vi "PLC_comm.vi"() -> ()   [LabVIEW 2017]
uses:
  <vilib>/DATA AHEAD/SP7/typedefs/PLC Type.ctl
  <vilib>/addons/database/Connection.llb/DB Tools Open Connec (String).vi
  Global/DATA LOG.vi
  <vilib>/DATA AHEAD/SP7/functions/write/write bool array.vi
  <vilib>/DATA AHEAD/SP7/functions/read/read bool array.vi
  <vilib>/DATA AHEAD/SP7/functions/read/read int array.vi
  <vilib>/DATA AHEAD/SP7/functions/read/read String.vi
  Global/Global 1.vi
  <vilib>/DATA AHEAD/SP7/functions/read/read real array.vi
  <vilib>/DATA AHEAD/SP7/functions/read/read Timeofday array.vi
  <vilib>/addons/database/NI_Database_API.lvlib
  <vilib>/DATA AHEAD/SP7/SP7.lvlib
panel:
  out "IP1 7":string
  out "PLC 7":bool
  out "IP1 6":string
  out "PLC 6":bool
  out "IP1 5":string
  out "PLC 5":bool
  out "PLC 4":bool
  out "PLC 3":bool
  out "PLC 2":bool
  out "PLC 1":bool
  out "IP1 4":string
  out "IP1 3":string
  out "IP1 2":string
  out "IP1":string
  in  "stop":bool
  out "error out":errorcluster
  in  "error in (no error)":errorcluster
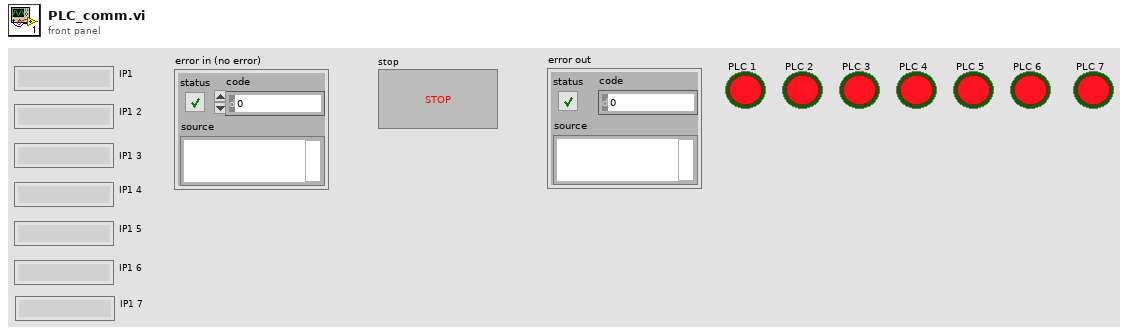
[diagram p1: front panel]
types:
  T1 = typedef "SP7.lvlib/PLC Type.ctl" = enum16{"S7 200", "S7 300/400", "S7 1200", "S7 1500", "LOGO!8"}
  T2 = typedef "NI_Database_API.lvlib/Conn ObjectReference.ctl" = refnum<k1>
  T3 = typedef "SP7.lvlib/S7 Connection.ctl" = cluster{"TCP Connection Ref":refnum<k5>, "IP address":string, "timeout ms":i32, "Connected?":bool, "PLC Type":T1, "Rack S7 400":u8, "Slot S7 400":u8, "PDU Size":u16, "connection semaphore":T4}
  T4 = typedef "Semaphore RefNum" = refnum<k1>
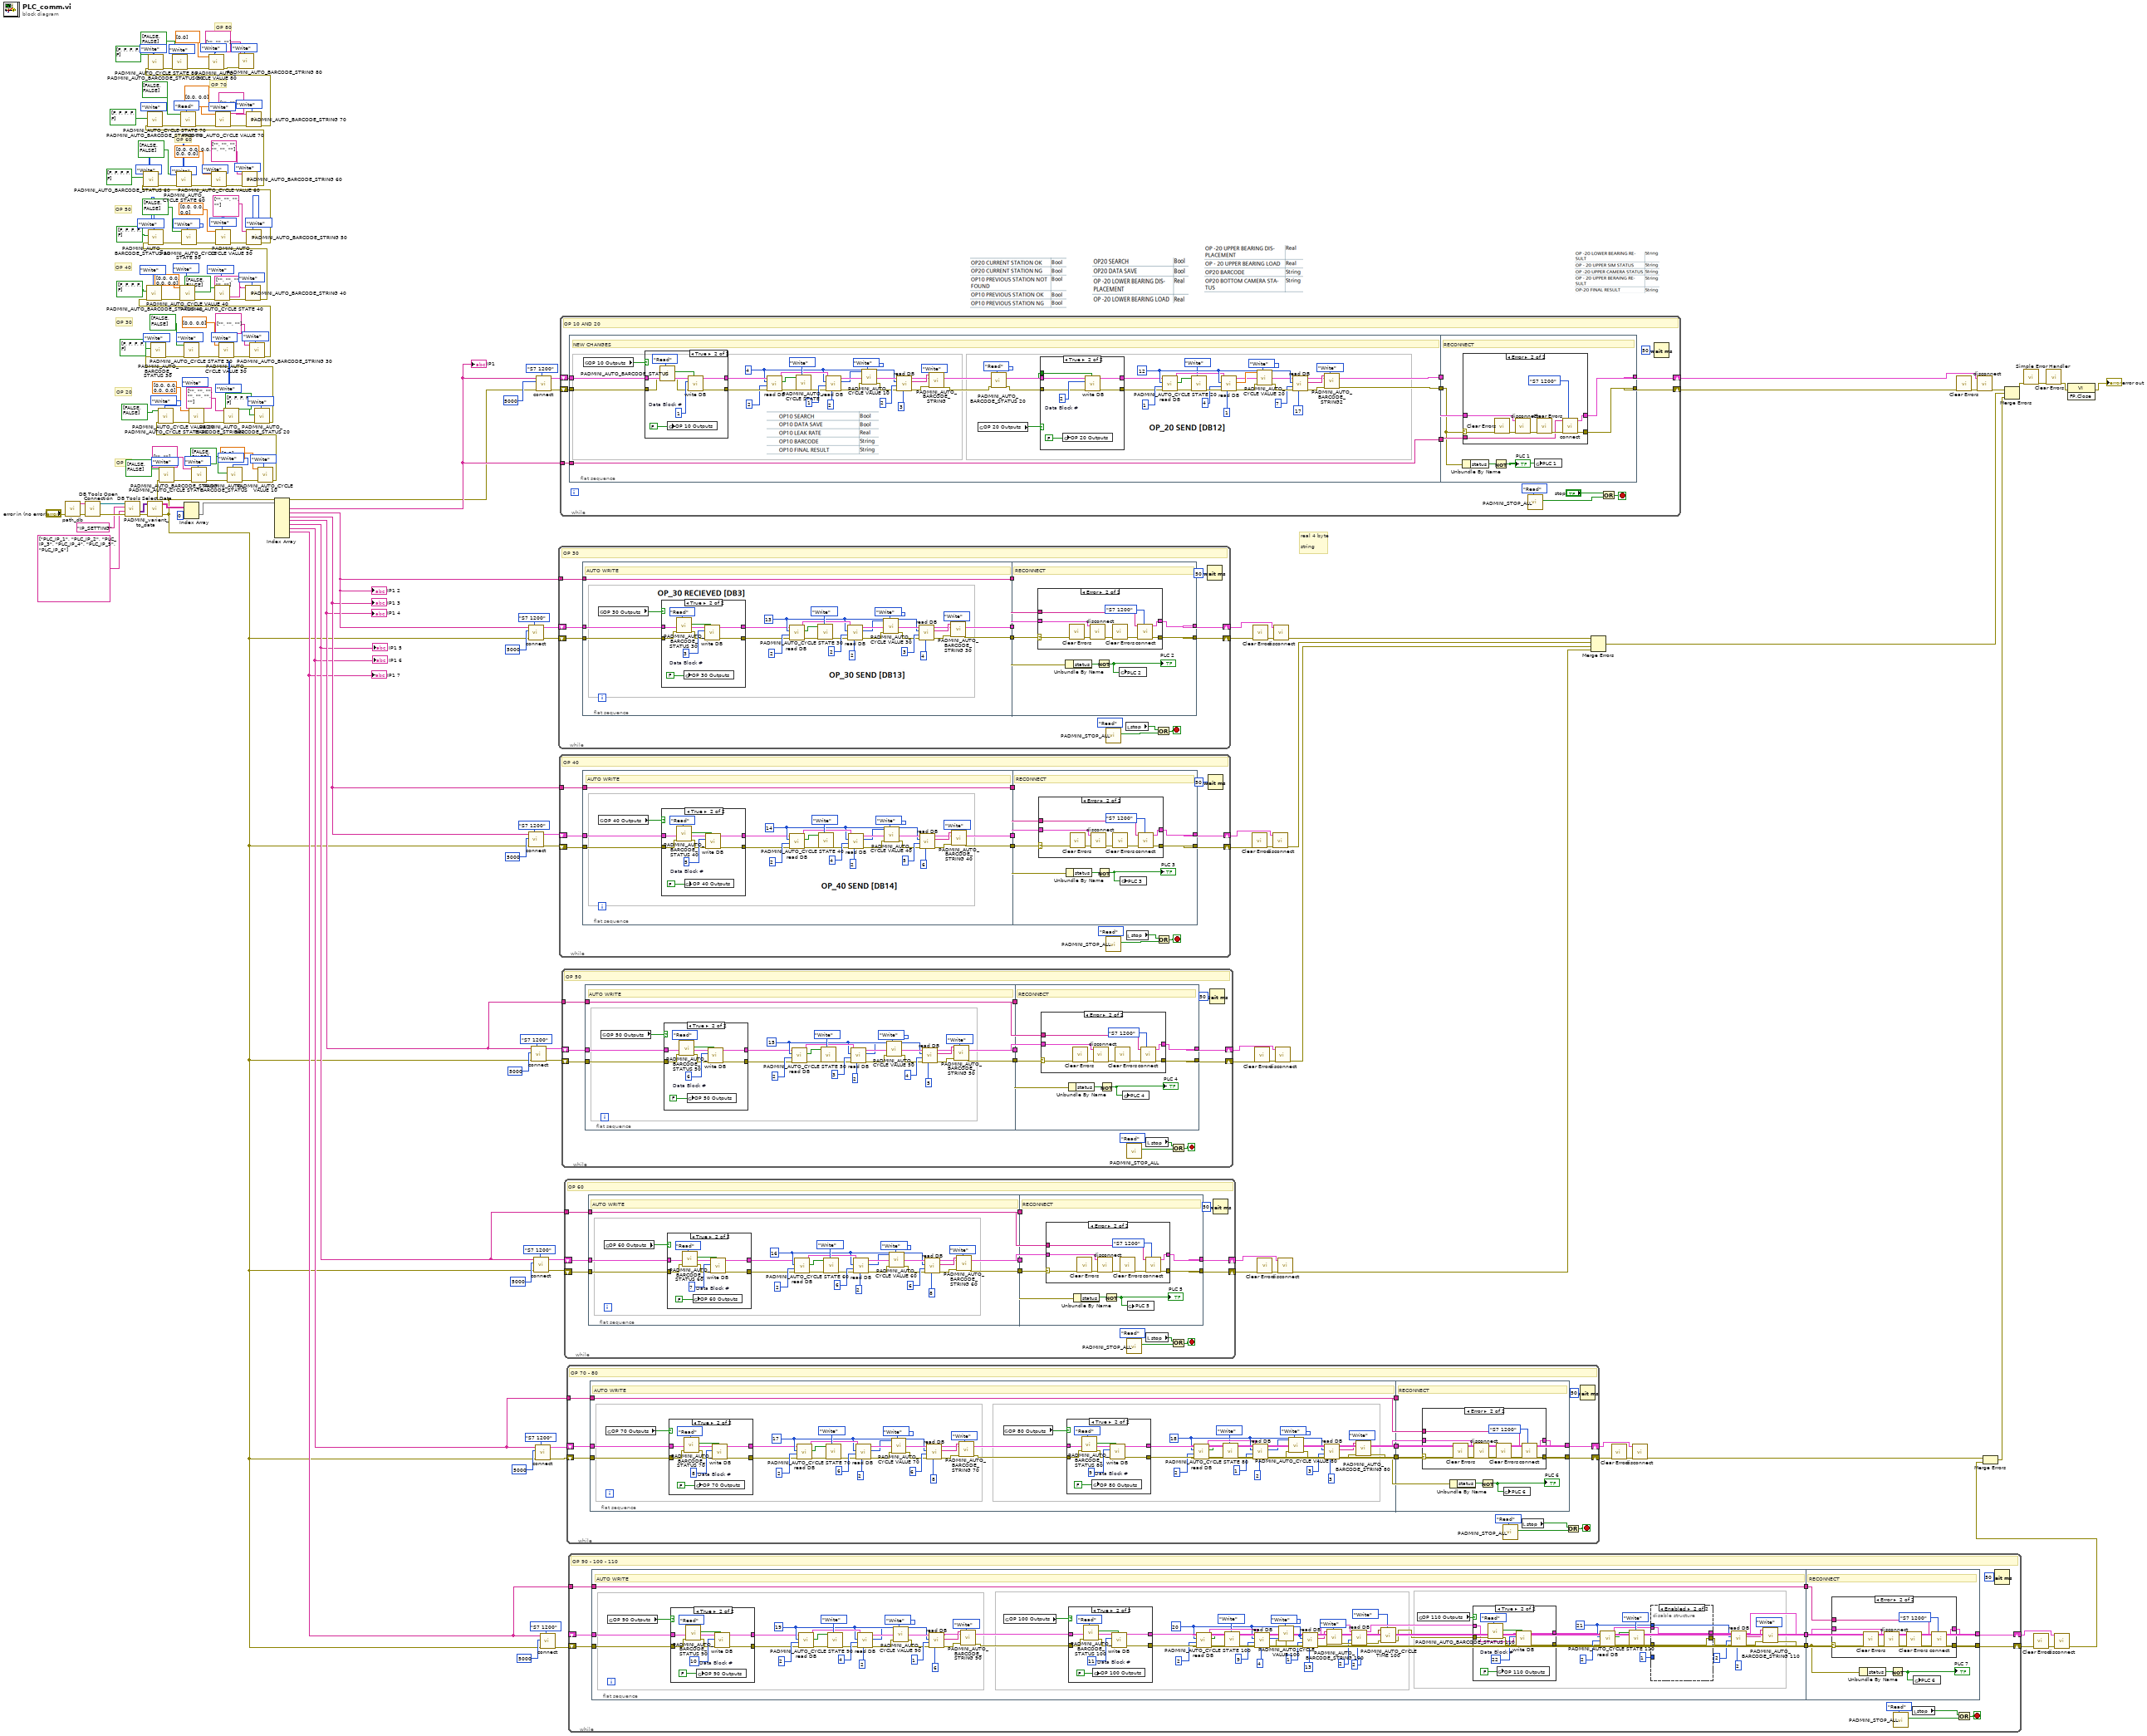
[diagram p0: block diagram]
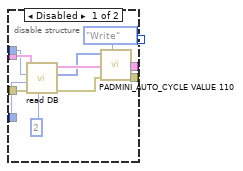
[diagram p2: hidden frame]
diagram:
  # "real 4 byte\n\nstring"
  # "OP 80"
  # "OP 70"
  # "OP 60"
  # "OP 50"
  # "OP 40"
  # "OP 30"
  # "OP 20"
  # "OP 10"
  n1 = call "path_db.vi"("error in"="error in (no error)") -> ("error out"=w171:errorcluster, "resulting string"=w176:string)  [unwired: 9 in]
  n2 = call-poly <vilib>:"DB Tools Open Connection.vi"("error in (no error)"=w171, "connection information"=w176) -> ("error out"=w175:errorcluster, "connection reference"=w174:T2)  [unwired: 6 in]
  n3 = call <vilib>:"DB Tools Select Data.vi"("error in (no error)"=w175, "columns"=string[] ["PLC_IP_1", "PLC_IP_2", "PLC_IP_3", "PLC_IP_4", "PLC_IP_5", "PLC_IP_6"], "table"="IP_SETTING", "connection reference"=w174) -> ("error out"=w173:errorcluster, "data"=w172:variant[][])  [unwired: 2 in, 1 out]
  n4 = call "PADMINI_varient_to_data.vi"("error in (no error)"=w173, "data"=w172) -> ("error out"=w7:errorcluster, "Array"=w167:string[][])  [unwired: 8 in]
  n5 = call "PADMINI_AUTO_CYCLE STATE.vi"("Enum"=enum16{"Read", "Write"}."Write", "error in (no error)"=w7, "Input"=bool[] [FALSE, FALSE]) -> ("error out"=w153:errorcluster)  [unwired: 7 in, 1 out]
  n6 = Index Array(array=w167, index (row)=0) -> (element=w166:string[])  [unwired: 1 in]
  n7 = call "PADMINI_AUTO_BARCODE_STRING.vi"("Enum"=enum16{"Read", "Write"}."Write", "error in (no error)"=w153, "Input"=string[] ["", ""]) -> ("error out"=w149:errorcluster)  [unwired: 7 in, 1 out]
  n8 = call "PADMINI_AUTO_BARCODE_STATUS.vi"("Enum"=enum16{"Read", "Write"}."Write", "error in (no error)"=w149, "I/P"=bool[] [FALSE, FALSE]) -> ("error out"=w147:errorcluster)  [unwired: 7 in, 1 out]
  n9 = call "PADMINI_AUTO_CYCLE VALUE 10.vi"("Enum"=enum16{"Read", "Write"}."Write", "error in (no error)"=w147, "Input"=dbl[] [0.0]) -> ("error out"=w141:errorcluster)  [unwired: 7 in, 1 out]
  n10 = call "PADMINI_AUTO_CYCLE STATE 20.vi"("Enum"=enum16{"Read", "Write"}."Write", "error in (no error)"=w141, "Input"=bool[] [FALSE, FALSE]) -> ("error out"=w139:errorcluster)  [unwired: 7 in, 1 out]
  n11 = call "PADMINI_AUTO_CYCLE VALUE 20.vi"("Enum"=enum16{"Read", "Write"}."Write", "error in (no error)"=w139, "Input"=dbl[] [0.0, 0.0, 0.0, 0.0]) -> ("error out"=w135:errorcluster)  [unwired: 7 in, 1 out]
  n12 = call "PADMINI_AUTO_BARCODE_STRING2.vi"("Enum"=enum16{"Read", "Write"}."Write", "error in (no error)"=w135, "Input"=string[] ["", "", "", "", "", "", ""]) -> ("error out"=w132:errorcluster)  [unwired: 7 in, 1 out]
  n13 = call "PADMINI_AUTO_BARCODE_STATUS 20.vi"("Enum"=enum16{"Read", "Write"}."Write", "error in (no error)"=w132, "I/P"=bool[] [FALSE, FALSE, FALSE, FALSE, FALSE]) -> ("error out"=w125:errorcluster)  [unwired: 7 in, 1 out]
  n14 = call "PADMINI_AUTO_BARCODE_STATUS 30.vi"("Enum"=enum16{"Read", "Write"}."Write", "error in (no error)"=w125, "I/P"=bool[] [FALSE, FALSE, FALSE, FALSE, FALSE]) -> ("error out"=w122:errorcluster)  [unwired: 7 in, 1 out]
  n15 = call "PADMINI_AUTO_CYCLE STATE 30.vi"("Enum"=enum16{"Read", "Write"}."Write", "error in (no error)"=w122, "Input"=bool[] [FALSE, FALSE]) -> ("error out"=w121:errorcluster)  [unwired: 7 in, 1 out]
  n16 = call "PADMINI_AUTO_CYCLE VALUE 30.vi"("Enum"=enum16{"Read", "Write"}."Write", "error in (no error)"=w121, "Input"=dbl[] [0.0, 0.0]) -> ("error out"=w117:errorcluster)  [unwired: 7 in, 1 out]
  n17 = call "PADMINI_AUTO_BARCODE_STRING 30.vi"("Enum"=enum16{"Read", "Write"}."Write", "error in (no error)"=w117, "Input"=string[] ["", "", ""]) -> ("error out"=w95:errorcluster)  [unwired: 7 in, 1 out]
  n18 = call "PADMINI_AUTO_BARCODE_STATUS 40.vi"("Enum"=enum16{"Read", "Write"}."Write", "error in (no error)"=w95, "I/P"=bool[] [FALSE, FALSE, FALSE, FALSE, FALSE]) -> ("error out"=w94:errorcluster)  [unwired: 7 in, 1 out]
  n19 = call "PADMINI_AUTO_CYCLE VALUE 40.vi"("Enum"=enum16{"Read", "Write"}."Write", "error in (no error)"=w94, "Input"=dbl[] [0.0, 0.0, 0.0, 0.0]) -> ("error out"=w93:errorcluster)  [unwired: 7 in, 1 out]
  n20 = call "PADMINI_AUTO_CYCLE STATE 40.vi"("Enum"=enum16{"Read", "Write"}."Write", "error in (no error)"=w93, "Input"=bool[] [FALSE, FALSE]) -> ("error out"=w92:errorcluster)  [unwired: 7 in, 1 out]
  n21 = call "PADMINI_AUTO_BARCODE_STRING 40.vi"("Enum"=enum16{"Read", "Write"}."Write", "error in (no error)"=w92, "Input"=string[] ["", "", "", "", ""]) -> ("error out"=w70:errorcluster)  [unwired: 7 in, 1 out]
  n22 = call "PADMINI_AUTO_BARCODE_STATUS 50.vi"("Enum"=enum16{"Read", "Write"}."Write", "error in (no error)"=w70, "I/P"=bool[] [FALSE, FALSE, FALSE, FALSE, FALSE]) -> ("error out"=w72:errorcluster)  [unwired: 7 in, 1 out]
  n23 = call "PADMINI_AUTO_CYCLE STATE 50.vi"("Enum"=enum16{"Read", "Write"}."Write", "error in (no error)"=w72, "Input"=bool[] [FALSE, FALSE]) -> ("error out"=w76:errorcluster)  [unwired: 7 in, 1 out]
  n24 = call "PADMINI_AUTO_CYCLE VALUE 50.vi"("Enum"=enum16{"Read", "Write"}."Write", "error in (no error)"=w76, "Input"=dbl[] [0.0, 0.0, 0.0]) -> ("error out"=w73:errorcluster)  [unwired: 7 in, 1 out]
  n25 = call "PADMINI_AUTO_BARCODE_STRING 50.vi"("Enum"=enum16{"Read", "Write"}."Write", "error in (no error)"=w73, "Input"=string[] ["", "", "", ""]) -> ("error out"=w44:errorcluster)  [unwired: 7 in, 1 out]
  n26 = call "PADMINI_AUTO_BARCODE_STATUS 60.vi"("Enum"=enum16{"Read", "Write"}."Write", "error in (no error)"=w44, "I/P"=bool[] [FALSE, FALSE, FALSE, FALSE, FALSE]) -> ("error out"=w50:errorcluster)  [unwired: 7 in, 1 out]
  n27 = call "PADMINI_AUTO_CYCLE STATE 60.vi"("Enum"=enum16{"Read", "Write"}."Write", "error in (no error)"=w50, "Input"=bool[] [FALSE, FALSE]) -> ("error out"=w52:errorcluster)  [unwired: 7 in, 1 out]
  n28 = call "PADMINI_AUTO_CYCLE VALUE 60.vi"("Enum"=enum16{"Read", "Write"}."Write", "error in (no error)"=w52, "Input"=dbl[] [0.0, 0.0, 0.0, 0.0, 0.0]) -> ("error out"=w55:errorcluster)  [unwired: 7 in, 1 out]
  n29 = call "PADMINI_AUTO_BARCODE_STRING 60.vi"("Enum"=enum16{"Read", "Write"}."Write", "error in (no error)"=w55, "Input"=string[] ["", "", "", "", "", ""]) -> ("error out"=w18:errorcluster)  [unwired: 7 in, 1 out]
  n30 = call "PADMINI_AUTO_BARCODE_STATUS 70.vi"("Enum"=enum16{"Read", "Write"}."Write", "error in (no error)"=w18, "I/P"=bool[] [FALSE, FALSE, FALSE, FALSE, FALSE]) -> ("error out"=w23:errorcluster)  [unwired: 7 in, 1 out]
  n31 = call "PADMINI_AUTO_CYCLE STATE 70.vi"("Enum"=enum16{"Read", "Write"}."Read", "error in (no error)"=w23, "Input"=bool[] [FALSE, FALSE]) -> ("error out"=w35:errorcluster)  [unwired: 7 in, 1 out]
  n32 = call "PADMINI_AUTO_CYCLE VALUE 70.vi"("Enum"=enum16{"Read", "Write"}."Write", "error in (no error)"=w35, "Input"=dbl[] [0.0, 0.0]) -> ("error out"=w32:errorcluster)  [unwired: 7 in, 1 out]
  n33 = call "PADMINI_AUTO_BARCODE_STRING 70.vi"("Enum"=enum16{"Read", "Write"}."Write", "error in (no error)"=w32, "Input"=string[] ["", ""]) -> ("error out"=w13:errorcluster)  [unwired: 7 in, 1 out]
  n34 = call "PADMINI_AUTO_BARCODE_STATUS 80.vi"("Enum"=enum16{"Read", "Write"}."Write", "error in (no error)"=w13, "I/P"=bool[] [FALSE, FALSE, FALSE, FALSE, FALSE]) -> ("error out"=w24:errorcluster)  [unwired: 7 in, 1 out]
  n35 = call "PADMINI_AUTO_CYCLE STATE 80.vi"("Enum"=enum16{"Read", "Write"}."Write", "error in (no error)"=w24, "Input"=bool[] [FALSE, FALSE]) -> ("error out"=w28:errorcluster)  [unwired: 7 in, 1 out]
  n36 = call "PADMINI_AUTO_CYCLE VALUE 80.vi"("Enum"=enum16{"Read", "Write"}."Write", "error in (no error)"=w28, "Input"=dbl[] [0.0]) -> ("error out"=w31:errorcluster)  [unwired: 7 in, 1 out]
  n37 = call "PADMINI_AUTO_BARCODE_STRING 80.vi"("Enum"=enum16{"Read", "Write"}."Write", "error in (no error)"=w31, "Input"=string[] ["", "", ""]) -> ()  [unwired: 7 in, 2 out]
  n38 = Index Array(array=w166) -> (element #1=w111:string, element #2=w112:string, element #3=w106:string, element #4=w80:string, element #5=w58:string, element #6=w9:string, element #7=w8:string)  [unwired: 8 in, 1 out]
  "IP1" <- w111
  "IP1 2" <- w112
  "IP1 3" <- w106
  "IP1 4" <- w80
  "IP1 5" <- w58
  "IP1 6" <- w9
  "IP1 7" <- w8
  n39 = call <vilib>:"connect.vi"("PLC Type"=PLC_Type."S7 1200" ("PLC Type 2"), "error in (no error)"=w7, "timeout [ms]"=5000 ("timeout [ms] 2"), "IP address"=w112) -> ("error out"=w129:errorcluster, "S7 Connection out"=w128:T3)  [unwired: 6 in]
  n40 = call <vilib>:"connect.vi"("PLC Type"=PLC_Type."S7 1200" ("PLC Type 2"), "error in (no error)"=w7, "timeout [ms]"=5000 ("timeout [ms] 2"), "IP address"=w106) -> ("error out"=w108:errorcluster, "S7 Connection out"=w107:T3)  [unwired: 6 in]
  n41 = call <vilib>:"connect.vi"("PLC Type"=PLC_Type."S7 1200" ("PLC Type 2"), "error in (no error)"=w7, "timeout [ms]"=5000 ("timeout [ms] 2"), "IP address"=w80) -> ("error out"=w83:errorcluster, "S7 Connection out"=w84:T3)  [unwired: 6 in]
  n42 = call <vilib>:"connect.vi"("PLC Type"=PLC_Type."S7 1200" ("PLC Type 2"), "error in (no error)"=w7, "timeout [ms]"=5000 ("timeout [ms] 2"), "IP address"=w58) -> ("error out"=w63:errorcluster, "S7 Connection out"=w62:T3)  [unwired: 6 in]
  n43 = call <vilib>:"connect.vi"("PLC Type"=PLC_Type."S7 1200" ("PLC Type 2"), "error in (no error)"=w7, "timeout [ms]"=5000 ("timeout [ms] 2"), "IP address"=w9) -> ("error out"=w41:errorcluster, "S7 Connection out"=w40:T3)  [unwired: 6 in]
  n44 = call <vilib>:"connect.vi"("PLC Type"=PLC_Type."S7 1200" ("PLC Type 2"), "error in (no error)"=w7, "timeout [ms]"=5000, "IP address"=w111) -> ("error out"=w157:errorcluster, "S7 Connection out"=w156:T3)  [unwired: 6 in]
  n45 = call <vilib>:"connect.vi"("PLC Type"=PLC_Type."S7 1200" ("PLC Type 2"), "error in (no error)"=w7, "timeout [ms]"=5000 ("timeout [ms] 2"), "IP address"=w8) -> ("error out"=w10:errorcluster)  [unwired: 6 in, 1 out]
  n46 = while {
    shift-right: [w179] -> w114
    shift-left: w128 -> [w189]
    shift-right: [w187] -> w113
    shift-left: w129 -> [w188]
    tunnel: w112 -> [w178]
    stop <- w181 stop-if-true
    # "OP 30"
    n47 = flat-sequence {
      tunnel: [w192] -> w185
      tunnel: [w191] -> w180
      tunnel: w188 -> [w216]
      tunnel: w189 -> [w215]
      tunnel: w178 -> [w190]
      tunnel: [w190] -> w177
      tunnel: [w230] -> w187
      tunnel: [w229] -> w179
      tunnel: w185 -> [w232]
      tunnel: w180 -> [w231]
      tunnel: w177 -> [w228]
      frame #0 {
        w205 = u16 13 ("Data Block #")
        # "AUTO WRITE"
        n48 = global read "DATA LOG.vi" "OP 30 Outputs"() -> (w214:bool)
        n49 = case shown="True" w214 {
          tunnel: w215 -> [w217 w226]
          tunnel: [w218 w225] -> w193
          tunnel: [w217 w224] -> w194
          tunnel: w216 -> [w218 w221]
          frame False {
          }
          frame True {
            w227 = u16 3  # Data Block #
            n50 = call "PADMINI_AUTO_BARCODE_STATUS 30.vi"("Enum"=enum16{"Read", "Write"}."Read", "error in (no error)"=w221) -> ("error out"=w220:errorcluster, "O/P"=w222:bool[])  [unwired: 8 in]
            n51 = global write "DATA LOG.vi" "OP 30 Outputs"(FALSE) -> ()
            n52 = call-poly <vilib>:"write DB.vi"("BOOL input array [byte]"=w222, "error in (no error)"=w220, "Data Block #"=w227, "S7 Connection in"=w226) -> ("error out"=w225:errorcluster, "S7 Connection out"=w224:T3)  [unwired: 4 in, 2 out]
          }
        }
        n53 = call-poly <vilib>:"read DB.vi"("error in (no error)"=w193, "Items # [byte]"=u16 2, "Data Block #"=w205, "S7 Connection in"=w194) -> ("error out"=w212:errorcluster, "BOOL result array  [byte]"=w210:bool[], "S7 Connection out"=w207:T3)  [unwired: 5 in]
        n54 = call "PADMINI_AUTO_CYCLE STATE 30.vi"("Enum"=enum16{"Read", "Write"}."Write", "error in (no error)"=w212, "Input"=w210) -> ("error out"=w208:errorcluster)  [unwired: 7 in, 1 out]
        n55 = call-poly <vilib>:"read DB.vi"("Item offset [byte]"=u32 2, "error in (no error)"=w208, "items #"=u16 2 ("Items # [byte]"), "Data Block #"=w205, "S7 Connection in"=w207) -> ("error out"=w197:errorcluster, "Int result array"=w195:i16[], "S7 Connection out"=w206:T3)  [unwired: 4 in]
        n56 = call "PADMINI_AUTO_CYCLE VALUE 30.vi"("Enum"=enum16{"Read", "Write"}."Write", "error in (no error)"=w197, "Input"=w195) -> ("error out"=w196:errorcluster)  [unwired: 7 in, 1 out]
        n57 = call-poly <vilib>:"read DB.vi"("Item offset [byte]"=u32 4, "error in (no error)"=w196, "items #"=u16 3 ("Items # [byte]"), "Data Block #"=w205, "S7 Connection in"=w206) -> ("error out"=w201:errorcluster, "STRING result Array"=w202:string[], "S7 Connection out"=w192:T3)  [unwired: 3 in, 1 out]
        n58 = call "PADMINI_AUTO_BARCODE_STRING 30.vi"("Enum"=enum16{"Read", "Write"}."Write", "error in (no error)"=w201, "Input"=w202) -> ("error out"=w191:errorcluster)  [unwired: 7 in, 1 out]
      }
      frame #1 {
        # "RECONNECT"
        n59 = case shown="Error" w231 {
          selector: w231 -> [w236 w244]
          tunnel: [w235 w241] -> w229
          tunnel: [w236 w242] -> w230
          tunnel: w232 -> [w235 w238]
          tunnel: w228 -> [_ w237]
          frame No Error {
          }
          frame Error {
            n60 = call <vilib>:"Clear Errors.vi"("error in (no error)"=w244) -> ("error out"=w245:errorcluster)  [unwired: 5 in, 1 out]
            n61 = call <vilib>:"disconnect.vi"("error in (no error)"=w245, "S7 Connection in"=w238) -> ("error out"=w243:errorcluster)  [unwired: 8 in, 1 out]
            n62 = call <vilib>:"Clear Errors.vi"("error in (no error)"=w243) -> ("error out"=w240:errorcluster)  [unwired: 5 in, 1 out]
            n63 = call <vilib>:"connect.vi"("PLC Type"=PLC_Type."S7 1200" ("PLC Type 2"), "error in (no error)"=w240, "IP address"=w237) -> ("error out"=w242:errorcluster, "S7 Connection out"=w241:T3)  [unwired: 7 in]
          }
        }
        n64 = Unbundle By Name(w231) -> ("status"=w234:bool)
        n65 = Not(x=w234) -> (.not. x?=w233:bool)
        "PLC 2" <- w233
        n66 = global write "Global 1.vi" "PLC 2"(w233) -> ()
      }
    }
    n67 = call "PADMINI_STOP_ALL.vi"("Enum"=enum16{"Read", "Write"}."Read") -> ("Boolean 2"=w183:bool)  [unwired: 9 in, 1 out]
    n68 = local read "stop"() -> (w182:bool)
    n69 = Or(x=w182, y=w183) -> (x .or. y?=w181:bool)
    n70 = Wait (ms)(milliseconds to wait=u32 50) -> ()  [unwired: 1 out]
  }
  n71 = while {
    shift-right: [w248] -> w103
    shift-left: w107 -> [w258]
    shift-right: [w256] -> w104
    shift-left: w108 -> [w257]
    tunnel: w106 -> [w247]
    stop <- w250 stop-if-true
    # "OP 40"
    n72 = flat-sequence {
      tunnel: [w261] -> w254
      tunnel: [w260] -> w249
      tunnel: w257 -> [w285]
      tunnel: w258 -> [w284]
      tunnel: w247 -> [w259]
      tunnel: [w259] -> w246
      tunnel: [w299] -> w256
      tunnel: [w298] -> w248
      tunnel: w254 -> [w301]
      tunnel: w249 -> [w300]
      tunnel: w246 -> [w297]
      frame #0 {
        w274 = u16 14 ("Data Block #")
        # "AUTO WRITE"
        n73 = global read "DATA LOG.vi" "OP 40 Outputs"() -> (w283:bool)
        n74 = case shown="True" w283 {
          tunnel: w284 -> [w286 w295]
          tunnel: [w287 w294] -> w262
          tunnel: [w286 w293] -> w263
          tunnel: w285 -> [w287 w290]
          frame False {
          }
          frame True {
            w296 = u16 5  # Data Block #
            n75 = call "PADMINI_AUTO_BARCODE_STATUS 40.vi"("Enum"=enum16{"Read", "Write"}."Read", "error in (no error)"=w290) -> ("error out"=w289:errorcluster, "O/P"=w291:bool[])  [unwired: 8 in]
            n76 = global write "DATA LOG.vi" "OP 40 Outputs"(FALSE) -> ()
            n77 = call-poly <vilib>:"write DB.vi"("BOOL input array [byte]"=w291, "error in (no error)"=w289, "Data Block #"=w296, "S7 Connection in"=w295) -> ("error out"=w294:errorcluster, "S7 Connection out"=w293:T3)  [unwired: 4 in, 2 out]
          }
        }
        n78 = call-poly <vilib>:"read DB.vi"("error in (no error)"=w262, "Items # [byte]"=u16 2, "Data Block #"=w274, "S7 Connection in"=w263) -> ("error out"=w281:errorcluster, "BOOL result array  [byte]"=w279:bool[], "S7 Connection out"=w276:T3)  [unwired: 5 in]
        n79 = call "PADMINI_AUTO_CYCLE STATE 40.vi"("Enum"=enum16{"Read", "Write"}."Write", "error in (no error)"=w281, "Input"=w279) -> ("error out"=w277:errorcluster)  [unwired: 7 in, 1 out]
        n80 = call-poly <vilib>:"read DB.vi"("Item offset [byte]"=u32 2, "error in (no error)"=w277, "items #"=u16 4 ("Items # [byte]"), "Data Block #"=w274, "S7 Connection in"=w276) -> ("error out"=w266:errorcluster, "Int result array"=w264:i16[], "S7 Connection out"=w275:T3)  [unwired: 4 in]
        n81 = call "PADMINI_AUTO_CYCLE VALUE 40.vi"("Enum"=enum16{"Read", "Write"}."Write", "error in (no error)"=w266, "Input"=w264) -> ("error out"=w265:errorcluster)  [unwired: 7 in, 1 out]
        n82 = call-poly <vilib>:"read DB.vi"("Item offset [byte]"=u32 6, "error in (no error)"=w265, "items #"=u16 5 ("Items # [byte]"), "Data Block #"=w274, "S7 Connection in"=w275) -> ("error out"=w270:errorcluster, "STRING result Array"=w271:string[], "S7 Connection out"=w261:T3)  [unwired: 3 in, 1 out]
        n83 = call "PADMINI_AUTO_BARCODE_STRING 40.vi"("Enum"=enum16{"Read", "Write"}."Write", "error in (no error)"=w270, "Input"=w271) -> ("error out"=w260:errorcluster)  [unwired: 7 in, 1 out]
      }
      frame #1 {
        # "RECONNECT"
        n84 = case shown="Error" w300 {
          selector: w300 -> [w305 w313]
          tunnel: [w304 w310] -> w298
          tunnel: [w305 w311] -> w299
          tunnel: w301 -> [w304 w307]
          tunnel: w297 -> [_ w306]
          frame No Error {
          }
          frame Error {
            n85 = call <vilib>:"Clear Errors.vi"("error in (no error)"=w313) -> ("error out"=w314:errorcluster)  [unwired: 5 in, 1 out]
            n86 = call <vilib>:"disconnect.vi"("error in (no error)"=w314, "S7 Connection in"=w307) -> ("error out"=w312:errorcluster)  [unwired: 8 in, 1 out]
            n87 = call <vilib>:"Clear Errors.vi"("error in (no error)"=w312) -> ("error out"=w309:errorcluster)  [unwired: 5 in, 1 out]
            n88 = call <vilib>:"connect.vi"("PLC Type"=PLC_Type."S7 1200" ("PLC Type 2"), "error in (no error)"=w309, "IP address"=w306) -> ("error out"=w311:errorcluster, "S7 Connection out"=w310:T3)  [unwired: 7 in]
          }
        }
        n89 = Unbundle By Name(w300) -> ("status"=w303:bool)
        n90 = Not(x=w303) -> (.not. x?=w302:bool)
        "PLC 3" <- w302
        n91 = global write "Global 1.vi" "PLC 3"(w302) -> ()
      }
    }
    n92 = call "PADMINI_STOP_ALL.vi"("Enum"=enum16{"Read", "Write"}."Read") -> ("Boolean 2"=w252:bool)  [unwired: 9 in, 1 out]
    n93 = local read "stop"() -> (w251:bool)
    n94 = Or(x=w251, y=w252) -> (x .or. y?=w250:bool)
    n95 = Wait (ms)(milliseconds to wait=u32 50) -> ()  [unwired: 1 out]
  }
  n96 = while {
    shift-right: [w317] -> w144
    shift-left: w156 -> [w327]
    shift-right: [w325] -> w160
    shift-left: w157 -> [w326]
    tunnel: w111 -> [w315]
    stop <- w320 stop-if-true
    # "OP 10 AND 20"
    n97 = flat-sequence {
      tunnel: [w330] -> w319
      tunnel: [w329] -> w318
      tunnel: w326 -> [w363]
      tunnel: w327 -> [w380]
      tunnel: [w328] -> w316
      tunnel: w315 -> [w328]
      tunnel: [w405] -> w325
      tunnel: [w404] -> w317
      tunnel: w319 -> [w406]
      tunnel: w318 -> [w402]
      tunnel: w316 -> [w403]
      frame #0 {
        w345 = u16 12 ("Data Block #")
        w370 = u16 4 ("Data Block #")
        # "NEW CHANGES"
        n98 = global read "DATA LOG.vi" "OP 10 Outputs"() -> (w362:bool)
        n99 = case shown="True" w362 {
          tunnel: w380 -> [w391 w400]
          tunnel: [w392 w399] -> w379
          tunnel: [w391 w398] -> w377
          tunnel: w363 -> [w392 w395]
          frame False {
          }
          frame True {
            w401 = u16 1  # Data Block #
            n100 = call "PADMINI_AUTO_BARCODE_STATUS.vi"("Enum"=enum16{"Read", "Write"}."Read", "error in (no error)"=w395) -> ("error out"=w394:errorcluster, "O/P"=w396:bool[])  [unwired: 8 in]
            n101 = global write "DATA LOG.vi" "OP 10 Outputs"(FALSE) -> ()
            n102 = call-poly <vilib>:"write DB.vi"("BOOL input array [byte]"=w396, "error in (no error)"=w394, "Data Block #"=w401, "S7 Connection in"=w400) -> ("error out"=w399:errorcluster, "S7 Connection out"=w398:T3)  [unwired: 4 in, 2 out]
          }
        }
        n103 = call-poly <vilib>:"read DB.vi"("error in (no error)"=w379, "Items # [byte]"=u16 2, "Data Block #"=w370, "S7 Connection in"=w377) -> ("error out"=w378:errorcluster, "BOOL result array  [byte]"=w375:bool[], "S7 Connection out"=w372:T3)  [unwired: 5 in]
        n104 = call "PADMINI_AUTO_CYCLE STATE.vi"("Enum"=enum16{"Read", "Write"}."Write", "error in (no error)"=w378, "Input"=w375) -> ("error out"=w373:errorcluster)  [unwired: 7 in, 1 out]
        n105 = call-poly <vilib>:"read DB.vi"("Item offset [byte]"=u32 2, "error in (no error)"=w373, "items #"=u16 1 ("Items # [byte]"), "Data Block #"=w370, "S7 Connection in"=w372) -> ("error out"=w360:errorcluster, "Int result array"=w358:i16[], "S7 Connection out"=w371:T3)  [unwired: 4 in]
        n106 = call "PADMINI_AUTO_CYCLE VALUE 10.vi"("Enum"=enum16{"Read", "Write"}."Write", "error in (no error)"=w360, "Input"=w358) -> ("error out"=w359:errorcluster)  [unwired: 7 in, 1 out]
        n107 = call-poly <vilib>:"read DB.vi"("Item offset [byte]"=u32 3, "error in (no error)"=w359, "items #"=u16 2 ("Items # [byte]"), "Data Block #"=w370, "S7 Connection in"=w371) -> ("error out"=w366:errorcluster, "STRING result Array"=w367:string[], "S7 Connection out"=w357:T3)  [unwired: 3 in, 1 out]
        n108 = call "PADMINI_AUTO_BARCODE_STRING.vi"("Enum"=enum16{"Read", "Write"}."Write", "error in (no error)"=w366, "Input"=w367) -> ("error out"=w333:errorcluster)  [unwired: 7 in, 1 out]
        n109 = global read "DATA LOG.vi" "OP 20 Outputs"() -> (w356:bool)
        n110 = call "PADMINI_AUTO_BARCODE_STATUS 20.vi"("Enum"=enum16{"Read", "Write"}."Read", "error in (no error)"=w333) -> ("error out"=w332:errorcluster, "O/P"=w331:bool[])  [unwired: 8 in]
        n111 = case shown="True" w356 {
          tunnel: w357 -> [w382 w386]
          tunnel: [w383 w389] -> w336
          tunnel: [w382 w388] -> w335
          tunnel: w332 -> [w383 w385]
          tunnel: w331 -> [_ w384]
          frame False {
          }
          frame True {
            w390 = u16 2  # Data Block #
            n112 = global write "DATA LOG.vi" "OP 20 Outputs"(FALSE) -> ()
            n113 = call-poly <vilib>:"write DB.vi"("BOOL input array [byte]"=w384, "error in (no error)"=w385, "Data Block #"=w390, "S7 Connection in"=w386) -> ("error out"=w389:errorcluster, "S7 Connection out"=w388:T3)  [unwired: 4 in, 2 out]
          }
        }
        n114 = call-poly <vilib>:"read DB.vi"("error in (no error)"=w336, "Items # [byte]"=u16 1, "Data Block #"=w345, "S7 Connection in"=w335) -> ("error out"=w338:errorcluster, "BOOL result array  [byte]"=w340:bool[], "S7 Connection out"=w343:T3)  [unwired: 5 in]
        n115 = call "PADMINI_AUTO_CYCLE STATE 20.vi"("Enum"=enum16{"Read", "Write"}."Write", "error in (no error)"=w338, "Input"=w340) -> ("error out"=w342:errorcluster)  [unwired: 7 in, 1 out]
        n116 = call-poly <vilib>:"read DB.vi"("Item offset [byte]"=u32 1, "error in (no error)"=w342, "items #"=u16 4 ("Items # [byte]"), "Data Block #"=w345, "S7 Connection in"=w343) -> ("error out"=w353:errorcluster, "REAL result array"=w355:sgl[], "S7 Connection out"=w344:T3)  [unwired: 4 in]
        n117 = call "PADMINI_AUTO_CYCLE VALUE 20.vi"("Enum"=enum16{"Read", "Write"}."Write", "error in (no error)"=w353, "Input"=w355) -> ("error out"=w354:errorcluster)  [unwired: 7 in, 1 out]
        n118 = call-poly <vilib>:"read DB.vi"("Item offset [byte]"=u32 17, "error in (no error)"=w354, "items #"=u16 7 ("Items # [byte]"), "Data Block #"=w345, "S7 Connection in"=w344) -> ("error out"=w349:errorcluster, "STRING result Array"=w348:string[], "S7 Connection out"=w330:T3)  [unwired: 3 in, 1 out]
        n119 = call "PADMINI_AUTO_BARCODE_STRING2.vi"("Enum"=enum16{"Read", "Write"}."Write", "error in (no error)"=w349, "Input"=w348) -> ("error out"=w329:errorcluster)  [unwired: 7 in, 1 out]
      }
      frame #1 {
        # "RECONNECT"
        n120 = Unbundle By Name(w402) -> ("status"=w408:bool)
        n121 = case shown="Error" w402 {
          selector: w402 -> [w410 w418]
          tunnel: [w409 w415] -> w404
          tunnel: [w410 w416] -> w405
          tunnel: w406 -> [w409 w412]
          tunnel: w403 -> [_ w411]
          frame No Error {
          }
          frame Error {
            n122 = call <vilib>:"Clear Errors.vi"("error in (no error)"=w418) -> ("error out"=w419:errorcluster)  [unwired: 5 in, 1 out]
            n123 = call <vilib>:"disconnect.vi"("error in (no error)"=w419, "S7 Connection in"=w412) -> ("error out"=w417:errorcluster)  [unwired: 8 in, 1 out]
            n124 = call <vilib>:"Clear Errors.vi"("error in (no error)"=w417) -> ("error out"=w414:errorcluster)  [unwired: 5 in, 1 out]
            n125 = call <vilib>:"connect.vi"("PLC Type"=PLC_Type."S7 1200" ("PLC Type 2"), "error in (no error)"=w414, "IP address"=w411) -> ("error out"=w416:errorcluster, "S7 Connection out"=w415:T3)  [unwired: 7 in]
          }
        }
        n126 = Not(x=w408) -> (.not. x?=w407:bool)
        "PLC 1" <- w407
        n127 = global write "Global 1.vi" "PLC 1"(w407) -> ()
      }
    }
    n128 = call "PADMINI_STOP_ALL.vi"("Enum"=enum16{"Read", "Write"}."Read") -> ("Boolean 2"=w322:bool)  [unwired: 9 in, 1 out]
    n129 = Or(x="stop", y=w322) -> (x .or. y?=w320:bool)
    n130 = Wait (ms)(milliseconds to wait=u32 50) -> ()  [unwired: 1 out]
  }
  n131 = while {
    shift-right: [w422] -> w87
    shift-left: w84 -> [w432]
    shift-right: [w430] -> w86
    shift-left: w83 -> [w431]
    tunnel: w80 -> [w421]
    stop <- w424 stop-if-true
    # "OP 50"
    n132 = flat-sequence {
      tunnel: [w435] -> w428
      tunnel: [w434] -> w423
      tunnel: w431 -> [w459]
      tunnel: w432 -> [w458]
      tunnel: w421 -> [w433]
      tunnel: [w433] -> w420
      tunnel: [w473] -> w430
      tunnel: [w472] -> w422
      tunnel: w428 -> [w475]
      tunnel: w423 -> [w474]
      tunnel: w420 -> [w471]
      frame #0 {
        w448 = u16 15 ("Data Block #")
        # "AUTO WRITE"
        n133 = global read "DATA LOG.vi" "OP 50 Outputs"() -> (w457:bool)
        n134 = case shown="True" w457 {
          tunnel: w458 -> [w460 w469]
          tunnel: [w461 w468] -> w436
          tunnel: [w460 w467] -> w437
          tunnel: w459 -> [w461 w464]
          frame False {
          }
          frame True {
            w470 = u16 6  # Data Block #
            n135 = call "PADMINI_AUTO_BARCODE_STATUS 50.vi"("Enum"=enum16{"Read", "Write"}."Read", "error in (no error)"=w464) -> ("error out"=w463:errorcluster, "O/P"=w465:bool[])  [unwired: 8 in]
            n136 = global write "DATA LOG.vi" "OP 50 Outputs"(FALSE) -> ()
            n137 = call-poly <vilib>:"write DB.vi"("BOOL input array [byte]"=w465, "error in (no error)"=w463, "Data Block #"=w470, "S7 Connection in"=w469) -> ("error out"=w468:errorcluster, "S7 Connection out"=w467:T3)  [unwired: 4 in, 2 out]
          }
        }
        n138 = call-poly <vilib>:"read DB.vi"("error in (no error)"=w436, "Items # [byte]"=u16 2, "Data Block #"=w448, "S7 Connection in"=w437) -> ("error out"=w455:errorcluster, "BOOL result array  [byte]"=w453:bool[], "S7 Connection out"=w450:T3)  [unwired: 5 in]
        n139 = call "PADMINI_AUTO_CYCLE STATE 50.vi"("Enum"=enum16{"Read", "Write"}."Write", "error in (no error)"=w455, "Input"=w453) -> ("error out"=w451:errorcluster)  [unwired: 7 in, 1 out]
        n140 = call-poly <vilib>:"read DB.vi"("Item offset [byte]"=u32 2, "error in (no error)"=w451, "items #"=u16 3 ("Items # [byte]"), "Data Block #"=w448, "S7 Connection in"=w450) -> ("error out"=w440:errorcluster, "Int result array"=w438:i16[], "S7 Connection out"=w449:T3)  [unwired: 4 in]
        n141 = call "PADMINI_AUTO_CYCLE VALUE 50.vi"("Enum"=enum16{"Read", "Write"}."Write", "error in (no error)"=w440, "Input"=w438) -> ("error out"=w439:errorcluster)  [unwired: 7 in, 1 out]
        n142 = call-poly <vilib>:"read DB.vi"("Item offset [byte]"=u32 5, "error in (no error)"=w439, "items #"=u16 4 ("Items # [byte]"), "Data Block #"=w448, "S7 Connection in"=w449) -> ("error out"=w444:errorcluster, "STRING result Array"=w445:string[], "S7 Connection out"=w435:T3)  [unwired: 3 in, 1 out]
        n143 = call "PADMINI_AUTO_BARCODE_STRING 50.vi"("Enum"=enum16{"Read", "Write"}."Write", "error in (no error)"=w444, "Input"=w445) -> ("error out"=w434:errorcluster)  [unwired: 7 in, 1 out]
      }
      frame #1 {
        # "RECONNECT"
        n144 = case shown="Error" w474 {
          selector: w474 -> [w479 w487]
          tunnel: [w478 w484] -> w472
          tunnel: [w479 w485] -> w473
          tunnel: w475 -> [w478 w481]
          tunnel: w471 -> [_ w480]
          frame No Error {
          }
          frame Error {
            n145 = call <vilib>:"Clear Errors.vi"("error in (no error)"=w487) -> ("error out"=w488:errorcluster)  [unwired: 5 in, 1 out]
            n146 = call <vilib>:"disconnect.vi"("error in (no error)"=w488, "S7 Connection in"=w481) -> ("error out"=w486:errorcluster)  [unwired: 8 in, 1 out]
            n147 = call <vilib>:"Clear Errors.vi"("error in (no error)"=w486) -> ("error out"=w483:errorcluster)  [unwired: 5 in, 1 out]
            n148 = call <vilib>:"connect.vi"("PLC Type"=PLC_Type."S7 1200" ("PLC Type 2"), "error in (no error)"=w483, "IP address"=w480) -> ("error out"=w485:errorcluster, "S7 Connection out"=w484:T3)  [unwired: 7 in]
          }
        }
        n149 = Unbundle By Name(w474) -> ("status"=w477:bool)
        n150 = Not(x=w477) -> (.not. x?=w476:bool)
        "PLC 4" <- w476
        n151 = global write "Global 1.vi" "PLC 4"(w476) -> ()
      }
    }
    n152 = call "PADMINI_STOP_ALL.vi"("Enum"=enum16{"Read", "Write"}."Read") -> ("Boolean 2"=w426:bool)  [unwired: 9 in, 1 out]
    n153 = local read "stop"() -> (w425:bool)
    n154 = Or(x=w425, y=w426) -> (x .or. y?=w424:bool)
    n155 = Wait (ms)(milliseconds to wait=u32 50) -> ()  [unwired: 1 out]
  }
  n156 = while {
    shift-right: [w491] -> w59
    shift-left: w62 -> [w501]
    shift-right: [w499] -> w60
    shift-left: w63 -> [w500]
    tunnel: w58 -> [w490]
    stop <- w493 stop-if-true
    # "OP 60"
    n157 = flat-sequence {
      tunnel: [w504] -> w497
      tunnel: [w503] -> w492
      tunnel: w500 -> [w528]
      tunnel: w501 -> [w527]
      tunnel: w490 -> [w502]
      tunnel: [w502] -> w489
      tunnel: [w542] -> w499
      tunnel: [w541] -> w491
      tunnel: w497 -> [w544]
      tunnel: w492 -> [w543]
      tunnel: w489 -> [w540]
      frame #0 {
        w517 = u16 16 ("Data Block #")
        # "AUTO WRITE"
        n158 = global read "DATA LOG.vi" "OP 60 Outputs"() -> (w526:bool)
        n159 = case shown="True" w526 {
          tunnel: w527 -> [w529 w538]
          tunnel: [w530 w537] -> w505
          tunnel: [w529 w536] -> w506
          tunnel: w528 -> [w530 w533]
          frame False {
          }
          frame True {
            w539 = u16 7  # Data Block #
            n160 = call "PADMINI_AUTO_BARCODE_STATUS 60.vi"("Enum"=enum16{"Read", "Write"}."Read", "error in (no error)"=w533) -> ("error out"=w532:errorcluster, "O/P"=w534:bool[])  [unwired: 8 in]
            n161 = global write "DATA LOG.vi" "OP 60 Outputs"(FALSE) -> ()
            n162 = call-poly <vilib>:"write DB.vi"("BOOL input array [byte]"=w534, "error in (no error)"=w532, "Data Block #"=w539, "S7 Connection in"=w538) -> ("error out"=w537:errorcluster, "S7 Connection out"=w536:T3)  [unwired: 4 in, 2 out]
          }
        }
        n163 = call-poly <vilib>:"read DB.vi"("error in (no error)"=w505, "Items # [byte]"=u16 2, "Data Block #"=w517, "S7 Connection in"=w506) -> ("error out"=w524:errorcluster, "BOOL result array  [byte]"=w522:bool[], "S7 Connection out"=w519:T3)  [unwired: 5 in]
        n164 = call "PADMINI_AUTO_CYCLE STATE 60.vi"("Enum"=enum16{"Read", "Write"}."Write", "error in (no error)"=w524, "Input"=w522) -> ("error out"=w520:errorcluster)  [unwired: 7 in, 1 out]
        n165 = call-poly <vilib>:"read DB.vi"("Item offset [byte]"=u32 2, "error in (no error)"=w520, "items #"=u16 6 ("Items # [byte]"), "Data Block #"=w517, "S7 Connection in"=w519) -> ("error out"=w509:errorcluster, "Int result array"=w507:i16[], "S7 Connection out"=w518:T3)  [unwired: 4 in]
        n166 = call "PADMINI_AUTO_CYCLE VALUE 60.vi"("Enum"=enum16{"Read", "Write"}."Write", "error in (no error)"=w509, "Input"=w507) -> ("error out"=w508:errorcluster)  [unwired: 7 in, 1 out]
        n167 = call-poly <vilib>:"read DB.vi"("Item offset [byte]"=u32 8, "error in (no error)"=w508, "items #"=u16 6 ("Items # [byte]"), "Data Block #"=w517, "S7 Connection in"=w518) -> ("error out"=w513:errorcluster, "STRING result Array"=w514:string[], "S7 Connection out"=w504:T3)  [unwired: 3 in, 1 out]
        n168 = call "PADMINI_AUTO_BARCODE_STRING 60.vi"("Enum"=enum16{"Read", "Write"}."Write", "error in (no error)"=w513, "Input"=w514) -> ("error out"=w503:errorcluster)  [unwired: 7 in, 1 out]
      }
      frame #1 {
        # "RECONNECT"
        n169 = case shown="Error" w543 {
          selector: w543 -> [w548 w556]
          tunnel: [w547 w553] -> w541
          tunnel: [w548 w554] -> w542
          tunnel: w544 -> [w547 w550]
          tunnel: w540 -> [_ w549]
          frame No Error {
          }
          frame Error {
            n170 = call <vilib>:"Clear Errors.vi"("error in (no error)"=w556) -> ("error out"=w557:errorcluster)  [unwired: 5 in, 1 out]
            n171 = call <vilib>:"disconnect.vi"("error in (no error)"=w557, "S7 Connection in"=w550) -> ("error out"=w555:errorcluster)  [unwired: 8 in, 1 out]
            n172 = call <vilib>:"Clear Errors.vi"("error in (no error)"=w555) -> ("error out"=w552:errorcluster)  [unwired: 5 in, 1 out]
            n173 = call <vilib>:"connect.vi"("PLC Type"=PLC_Type."S7 1200" ("PLC Type 2"), "error in (no error)"=w552, "IP address"=w549) -> ("error out"=w554:errorcluster, "S7 Connection out"=w553:T3)  [unwired: 7 in]
          }
        }
        n174 = Unbundle By Name(w543) -> ("status"=w546:bool)
        n175 = Not(x=w546) -> (.not. x?=w545:bool)
        "PLC 5" <- w545
        n176 = global write "Global 1.vi" "PLC 5"(w545) -> ()
      }
    }
    n177 = call "PADMINI_STOP_ALL.vi"("Enum"=enum16{"Read", "Write"}."Read") -> ("Boolean 2"=w495:bool)  [unwired: 9 in, 1 out]
    n178 = local read "stop"() -> (w494:bool)
    n179 = Or(x=w494, y=w495) -> (x .or. y?=w493:bool)
    n180 = Wait (ms)(milliseconds to wait=u32 50) -> ()  [unwired: 1 out]
  }
  n181 = while {
    shift-right: [w560] -> w37
    shift-left: w40 -> [w570]
    shift-right: [w568] -> w38
    shift-left: w41 -> [w569]
    tunnel: w9 -> [w559]
    stop <- w562 stop-if-true
    # "OP 70 - 80"
    n182 = flat-sequence {
      tunnel: [w571] -> w566
      tunnel: [w572] -> w561
      tunnel: w569 -> [w621]
      tunnel: w570 -> [w620]
      tunnel: w559 -> [w597]
      tunnel: [w597] -> w558
      tunnel: [w646] -> w568
      tunnel: [w645] -> w560
      tunnel: w566 -> [w648]
      tunnel: w561 -> [w647]
      tunnel: w558 -> [w644]
      frame #0 {
        w584 = u16 18 ("Data Block #")
        w610 = u16 17 ("Data Block #")
        # "AUTO WRITE"
        n183 = global read "DATA LOG.vi" "OP 70 Outputs"() -> (w619:bool)
        n184 = case shown="True" w619 {
          tunnel: w620 -> [w633 w642]
          tunnel: [w634 w641] -> w598
          tunnel: [w633 w640] -> w599
          tunnel: w621 -> [w634 w637]
          frame False {
          }
          frame True {
            w643 = u16 8  # Data Block #
            n185 = call "PADMINI_AUTO_BARCODE_STATUS 70.vi"("Enum"=enum16{"Read", "Write"}."Read", "error in (no error)"=w637) -> ("error out"=w636:errorcluster, "O/P"=w638:bool[])  [unwired: 8 in]
            n186 = global write "DATA LOG.vi" "OP 70 Outputs"(FALSE) -> ()
            n187 = call-poly <vilib>:"write DB.vi"("BOOL input array [byte]"=w638, "error in (no error)"=w636, "Data Block #"=w643, "S7 Connection in"=w642) -> ("error out"=w641:errorcluster, "S7 Connection out"=w640:T3)  [unwired: 4 in, 2 out]
          }
        }
        n188 = call-poly <vilib>:"read DB.vi"("error in (no error)"=w598, "Items # [byte]"=u16 2, "Data Block #"=w610, "S7 Connection in"=w599) -> ("error out"=w617:errorcluster, "BOOL result array  [byte]"=w615:bool[], "S7 Connection out"=w612:T3)  [unwired: 5 in]
        n189 = call "PADMINI_AUTO_CYCLE STATE 70.vi"("Enum"=enum16{"Read", "Write"}."Write", "error in (no error)"=w617, "Input"=w615) -> ("error out"=w613:errorcluster)  [unwired: 7 in, 1 out]
        n190 = call-poly <vilib>:"read DB.vi"("Item offset [byte]"=u32 2, "error in (no error)"=w613, "items #"=u16 6 ("Items # [byte]"), "Data Block #"=w610, "S7 Connection in"=w612) -> ("error out"=w602:errorcluster, "Int result array"=w600:i16[], "S7 Connection out"=w611:T3)  [unwired: 4 in]
        n191 = call "PADMINI_AUTO_CYCLE VALUE 70.vi"("Enum"=enum16{"Read", "Write"}."Write", "error in (no error)"=w602, "Input"=w600) -> ("error out"=w601:errorcluster)  [unwired: 7 in, 1 out]
        n192 = call-poly <vilib>:"read DB.vi"("Item offset [byte]"=u32 8, "error in (no error)"=w601, "items #"=u16 6 ("Items # [byte]"), "Data Block #"=w610, "S7 Connection in"=w611) -> ("error out"=w606:errorcluster, "STRING result Array"=w607:string[], "S7 Connection out"=w574:T3)  [unwired: 3 in, 1 out]
        n193 = call "PADMINI_AUTO_BARCODE_STRING 70.vi"("Enum"=enum16{"Read", "Write"}."Write", "error in (no error)"=w606, "Input"=w607) -> ("error out"=w573:errorcluster)  [unwired: 7 in, 1 out]
        n194 = global read "DATA LOG.vi" "OP 80 Outputs"() -> (w575:bool)
        n195 = case shown="True" w575 {
          tunnel: w574 -> [w622 w631]
          tunnel: [w623 w630] -> w596
          tunnel: [w622 w629] -> w595
          tunnel: w573 -> [w623 w626]
          frame False {
          }
          frame True {
            w632 = u16 9  # Data Block #
            n196 = call "PADMINI_AUTO_BARCODE_STATUS 80.vi"("Enum"=enum16{"Read", "Write"}."Read", "error in (no error)"=w626) -> ("error out"=w625:errorcluster, "O/P"=w627:bool[])  [unwired: 8 in]
            n197 = global write "DATA LOG.vi" "OP 80 Outputs"(FALSE) -> ()
            n198 = call-poly <vilib>:"write DB.vi"("BOOL input array [byte]"=w627, "error in (no error)"=w625, "Data Block #"=w632, "S7 Connection in"=w631) -> ("error out"=w630:errorcluster, "S7 Connection out"=w629:T3)  [unwired: 4 in, 2 out]
          }
        }
        n199 = call-poly <vilib>:"read DB.vi"("error in (no error)"=w596, "Items # [byte]"=u16 2, "Data Block #"=w584, "S7 Connection in"=w595) -> ("error out"=w577:errorcluster, "BOOL result array  [byte]"=w579:bool[], "S7 Connection out"=w582:T3)  [unwired: 5 in]
        n200 = call "PADMINI_AUTO_CYCLE STATE 80.vi"("Enum"=enum16{"Read", "Write"}."Write", "error in (no error)"=w577, "Input"=w579) -> ("error out"=w581:errorcluster)  [unwired: 7 in, 1 out]
        n201 = call-poly <vilib>:"read DB.vi"("Item offset [byte]"=u32 2, "error in (no error)"=w581, "items #"=u16 1 ("Items # [byte]"), "Data Block #"=w584, "S7 Connection in"=w582) -> ("error out"=w592:errorcluster, "Int result array"=w594:i16[], "S7 Connection out"=w583:T3)  [unwired: 4 in]
        n202 = call "PADMINI_AUTO_CYCLE VALUE 80.vi"("Enum"=enum16{"Read", "Write"}."Write", "error in (no error)"=w592, "Input"=w594) -> ("error out"=w593:errorcluster)  [unwired: 7 in, 1 out]
        n203 = call-poly <vilib>:"read DB.vi"("Item offset [byte]"=u32 3, "error in (no error)"=w593, "items #"=u16 3 ("Items # [byte]"), "Data Block #"=w584, "S7 Connection in"=w583) -> ("error out"=w588:errorcluster, "STRING result Array"=w587:string[], "S7 Connection out"=w571:T3)  [unwired: 3 in, 1 out]
        n204 = call "PADMINI_AUTO_BARCODE_STRING 80.vi"("Enum"=enum16{"Read", "Write"}."Write", "error in (no error)"=w588, "Input"=w587) -> ("error out"=w572:errorcluster)  [unwired: 7 in, 1 out]
      }
      frame #1 {
        # "RECONNECT"
        n205 = case shown="Error" w647 {
          selector: w647 -> [w652 w660]
          tunnel: [w651 w657] -> w645
          tunnel: [w652 w658] -> w646
          tunnel: w648 -> [w651 w654]
          tunnel: w644 -> [_ w653]
          frame No Error {
          }
          frame Error {
            n206 = call <vilib>:"Clear Errors.vi"("error in (no error)"=w660) -> ("error out"=w661:errorcluster)  [unwired: 5 in, 1 out]
            n207 = call <vilib>:"disconnect.vi"("error in (no error)"=w661, "S7 Connection in"=w654) -> ("error out"=w659:errorcluster)  [unwired: 8 in, 1 out]
            n208 = call <vilib>:"Clear Errors.vi"("error in (no error)"=w659) -> ("error out"=w656:errorcluster)  [unwired: 5 in, 1 out]
            n209 = call <vilib>:"connect.vi"("PLC Type"=PLC_Type."S7 1200" ("PLC Type 2"), "error in (no error)"=w656, "IP address"=w653) -> ("error out"=w658:errorcluster, "S7 Connection out"=w657:T3)  [unwired: 7 in]
          }
        }
        n210 = Unbundle By Name(w647) -> ("status"=w650:bool)
        n211 = Not(x=w650) -> (.not. x?=w649:bool)
        "PLC 6" <- w649
        n212 = global write "Global 1.vi" "PLC 6"(w649) -> ()
      }
    }
    n213 = call "PADMINI_STOP_ALL.vi"("Enum"=enum16{"Read", "Write"}."Read") -> ("Boolean 2"=w564:bool)  [unwired: 9 in, 1 out]
    n214 = local read "stop"() -> (w563:bool)
    n215 = Or(x=w563, y=w564) -> (x .or. y?=w562:bool)
    n216 = Wait (ms)(milliseconds to wait=u32 50) -> ()  [unwired: 1 out]
  }
  n217 = while {
    shift-right: [w664] -> w4
    shift-left: _ -> [w674]
    shift-right: [w672] -> w5
    shift-left: w10 -> [w673]
    tunnel: w8 -> [w663]
    stop <- w666 stop-if-true
    # "OP 90 - 100 - 110"
    n218 = flat-sequence {
      tunnel: [w685] -> w670
      tunnel: [w686] -> w665
      tunnel: w673 -> [w752]
      tunnel: w674 -> [w751]
      tunnel: w663 -> [w728]
      tunnel: [w728] -> w662
      tunnel: [w800] -> w672
      tunnel: [w799] -> w664
      tunnel: w670 -> [w802]
      tunnel: w665 -> [w801]
      tunnel: w662 -> [w798]
      frame #0 {
        w695 = u16 21 ("Data Block #")
        w679 = u16 20 ("Data Block #")
        w741 = u16 19 ("Data Block #")
        # "AUTO WRITE"
        n219 = global read "DATA LOG.vi" "OP 90 Outputs"() -> (w750:bool)
        n220 = case shown="True" w750 {
          tunnel: w751 -> [w787 w796]
          tunnel: [w788 w795] -> w729
          tunnel: [w787 w794] -> w730
          tunnel: w752 -> [w788 w791]
          frame False {
          }
          frame True {
            w797 = u16 10  # Data Block #
            n221 = call "PADMINI_AUTO_BARCODE_STATUS 90.vi"("Enum"=enum16{"Read", "Write"}."Read", "error in (no error)"=w791) -> ("error out"=w790:errorcluster, "O/P"=w792:bool[])  [unwired: 8 in]
            n222 = global write "DATA LOG.vi" "OP 90 Outputs"(FALSE) -> ()
            n223 = call-poly <vilib>:"write DB.vi"("BOOL input array [byte]"=w792, "error in (no error)"=w790, "Data Block #"=w797, "S7 Connection in"=w796) -> ("error out"=w795:errorcluster, "S7 Connection out"=w794:T3)  [unwired: 4 in, 2 out]
          }
        }
        n224 = call-poly <vilib>:"read DB.vi"("error in (no error)"=w729, "Items # [byte]"=u16 2, "Data Block #"=w741, "S7 Connection in"=w730) -> ("error out"=w748:errorcluster, "BOOL result array  [byte]"=w746:bool[], "S7 Connection out"=w743:T3)  [unwired: 5 in]
        n225 = call "PADMINI_AUTO_CYCLE STATE 90.vi"("Enum"=enum16{"Read", "Write"}."Write", "error in (no error)"=w748, "Input"=w746) -> ("error out"=w744:errorcluster)  [unwired: 7 in, 1 out]
        n226 = call-poly <vilib>:"read DB.vi"("Item offset [byte]"=u32 2, "error in (no error)"=w744, "items #"=u16 4 ("Items # [byte]"), "Data Block #"=w741, "S7 Connection in"=w743) -> ("error out"=w733:errorcluster, "Int result array"=w731:i16[], "S7 Connection out"=w742:T3)  [unwired: 4 in]
        n227 = call "PADMINI_AUTO_CYCLE VALUE 90.vi"("Enum"=enum16{"Read", "Write"}."Write", "error in (no error)"=w733, "Input"=w731) -> ("error out"=w732:errorcluster)  [unwired: 7 in, 1 out]
        n228 = call-poly <vilib>:"read DB.vi"("Item offset [byte]"=u32 6, "error in (no error)"=w732, "items #"=u16 1 ("Items # [byte]"), "Data Block #"=w741, "S7 Connection in"=w742) -> ("error out"=w737:errorcluster, "STRING result Array"=w738:string[], "S7 Connection out"=w706:T3)  [unwired: 3 in, 1 out]
        n229 = call "PADMINI_AUTO_BARCODE_STRING 90.vi"("Enum"=enum16{"Read", "Write"}."Write", "error in (no error)"=w737, "Input"=w738) -> ("error out"=w705:errorcluster)  [unwired: 7 in, 1 out]
        n230 = global read "DATA LOG.vi" "OP 100 Outputs"() -> (w707:bool)
        n231 = case shown="True" w707 {
          tunnel: w706 -> [w776 w785]
          tunnel: [w777 w784] -> w727
          tunnel: [w776 w783] -> w726
          tunnel: w705 -> [w777 w780]
          frame False {
          }
          frame True {
            w786 = u16 11  # Data Block #
            n232 = call "PADMINI_AUTO_BARCODE_STATUS 100.vi"("Enum"=enum16{"Read", "Write"}."Read", "error in (no error)"=w780) -> ("error out"=w779:errorcluster, "O/P"=w781:bool[])  [unwired: 8 in]
            n233 = global write "DATA LOG.vi" "OP 100 Outputs"(FALSE) -> ()
            n234 = call-poly <vilib>:"write DB.vi"("BOOL input array [byte]"=w781, "error in (no error)"=w779, "Data Block #"=w786, "S7 Connection in"=w785) -> ("error out"=w784:errorcluster, "S7 Connection out"=w783:T3)  [unwired: 4 in, 2 out]
          }
        }
        n235 = call-poly <vilib>:"read DB.vi"("error in (no error)"=w727, "Items # [byte]"=u16 2, "Data Block #"=w679, "S7 Connection in"=w726) -> ("error out"=w709:errorcluster, "BOOL result array  [byte]"=w711:bool[], "S7 Connection out"=w714:T3)  [unwired: 5 in]
        n236 = call "PADMINI_AUTO_CYCLE STATE 100.vi"("Enum"=enum16{"Read", "Write"}."Write", "error in (no error)"=w709, "Input"=w711) -> ("error out"=w713:errorcluster)  [unwired: 7 in, 1 out]
        n237 = call-poly <vilib>:"read DB.vi"("Item offset [byte]"=u32 4, "error in (no error)"=w713, "items #"=u16 9 ("Items # [byte]"), "Data Block #"=w679, "S7 Connection in"=w714) -> ("error out"=w723:errorcluster, "Int result array"=w725:i16[], "S7 Connection out"=w715:T3)  [unwired: 4 in]
        n238 = call "PADMINI_AUTO_CYCLE VALUE 100.vi"("Enum"=enum16{"Read", "Write"}."Write", "error in (no error)"=w723, "Input"=w725) -> ("error out"=w724:errorcluster)  [unwired: 7 in, 1 out]
        n239 = call-poly <vilib>:"read DB.vi"("Item offset [byte]"=u32 13, "error in (no error)"=w724, "items #"=u16 1 ("Items # [byte]"), "Data Block #"=w679, "S7 Connection in"=w715) -> ("error out"=w719:errorcluster, "STRING result Array"=w718:string[], "S7 Connection out"=w683:T3)  [unwired: 3 in, 1 out]
        n240 = call "PADMINI_AUTO_BARCODE_STRING 100.vi"("Enum"=enum16{"Read", "Write"}."Write", "error in (no error)"=w719, "Input"=w718) -> ("error out"=w684:errorcluster)  [unwired: 7 in, 1 out]
        n241 = call-poly <vilib>:"read DB.vi"("Item offset [byte]"=u32 2, "error in (no error)"=w684, "items #"=u32 2 ("Item offset [byte]"), "Data Block #"=w679, "S7 Connection in"=w683) -> ("error out"=w677:errorcluster, "Time of Day result array"=w675:timestamp[], "S7 Connection out"=w682:T3)  [unwired: 4 in]
        n242 = call "PADMINI_AUTO_CYCLE TIME 100.vi"("Enum"=enum16{"Read", "Write"}."Write", "error in (no error)"=w677, "Time of Day result array in"=w675) -> ("error out"=w676:errorcluster)  [unwired: 7 in, 1 out]
        n243 = global read "DATA LOG.vi" "OP 110 Outputs"() -> (w704:bool)
        n244 = case shown="True" w704 {
          tunnel: [w765 w774] -> w687
          tunnel: [w766 w773] -> w688
          tunnel: w676 -> [w765 w768]
          tunnel: w682 -> [w766 w767]
          frame False {
          }
          frame True {
            w775 = u16 22  # Data Block #
            n245 = call "PADMINI_AUTO_BARCODE_STATUS 110.vi"("Enum"=enum16{"Read", "Write"}."Read", "error in (no error)"=w768) -> ("error out"=w770:errorcluster, "O/P"=w771:bool[])  [unwired: 8 in]
            n246 = global write "DATA LOG.vi" "OP 110 Outputs"(FALSE) -> ()
            n247 = call-poly <vilib>:"write DB.vi"("BOOL input array [byte]"=w771, "error in (no error)"=w770, "Data Block #"=w775, "S7 Connection in"=w767) -> ("error out"=w774:errorcluster, "S7 Connection out"=w773:T3)  [unwired: 4 in, 2 out]
          }
        }
        n248 = call-poly <vilib>:"read DB.vi"("error in (no error)"=w687, "Items # [byte]"=u16 2, "Data Block #"=w695, "S7 Connection in"=w688) -> ("error out"=w702:errorcluster, "BOOL result array  [byte]"=w700:bool[], "S7 Connection out"=w697:T3)  [unwired: 5 in]
        n249 = call "PADMINI_AUTO_CYCLE STATE 110.vi"("Enum"=enum16{"Read", "Write"}."Write", "error in (no error)"=w702, "Input"=w700) -> ("error out"=w698:errorcluster)  [unwired: 7 in, 1 out]
        n250 = disable-structure shown="Enabled" {
          disable-tunnel: u16 1 ("Items # [byte]") -> [w762 _]
          disable-tunnel: w698 -> [w761 w763]
          disable-tunnel: w697 -> [w760 w764]
          disable-tunnel: [w759 w764] -> w696
          disable-tunnel: w695 -> [w758 _]
          disable-tunnel: [w754 w763] -> w689
          frame Disabled {
            n251 = call-poly <vilib>:"read DB.vi"("Item offset [byte]"=u32 2, "error in (no error)"=w761, "items #"=w762, "Data Block #"=w758, "S7 Connection in"=w760) -> ("error out"=w755:errorcluster, "Int result array"=w753:i16[], "S7 Connection out"=w759:T3)  [unwired: 4 in]
            n252 = call "PADMINI_AUTO_CYCLE VALUE 110.vi"("Enum"=enum16{"Read", "Write"}."Write", "error in (no error)"=w755, "Input"=w753) -> ("error out"=w754:errorcluster)  [unwired: 7 in, 1 out]
          }
          frame Enabled {
          }
        }
        n253 = call-poly <vilib>:"read DB.vi"("Item offset [byte]"=u32 2, "error in (no error)"=w689, "items #"=u16 2 ("Items # [byte]"), "Data Block #"=w695, "S7 Connection in"=w696) -> ("error out"=w691:errorcluster, "STRING result Array"=w692:string[], "S7 Connection out"=w685:T3)  [unwired: 3 in, 1 out]
        n254 = call "PADMINI_AUTO_BARCODE_STRING 110.vi"("Enum"=enum16{"Read", "Write"}."Write", "error in (no error)"=w691, "Input"=w692) -> ("error out"=w686:errorcluster)  [unwired: 7 in, 1 out]
      }
      frame #1 {
        # "RECONNECT"
        n255 = case shown="Error" w801 {
          selector: w801 -> [w806 w814]
          tunnel: [w805 w811] -> w799
          tunnel: [w806 w812] -> w800
          tunnel: w802 -> [w805 w808]
          tunnel: w798 -> [_ w807]
          frame No Error {
          }
          frame Error {
            n256 = call <vilib>:"Clear Errors.vi"("error in (no error)"=w814) -> ("error out"=w815:errorcluster)  [unwired: 5 in, 1 out]
            n257 = call <vilib>:"disconnect.vi"("error in (no error)"=w815, "S7 Connection in"=w808) -> ("error out"=w813:errorcluster)  [unwired: 8 in, 1 out]
            n258 = call <vilib>:"Clear Errors.vi"("error in (no error)"=w813) -> ("error out"=w810:errorcluster)  [unwired: 5 in, 1 out]
            n259 = call <vilib>:"connect.vi"("PLC Type"=PLC_Type."S7 1200" ("PLC Type 2"), "error in (no error)"=w810, "IP address"=w807) -> ("error out"=w812:errorcluster, "S7 Connection out"=w811:T3)  [unwired: 7 in]
          }
        }
        n260 = Unbundle By Name(w801) -> ("status"=w804:bool)
        n261 = Not(x=w804) -> (.not. x?=w803:bool)
        "PLC 7" <- w803
        n262 = global write "Global 1.vi" "PLC 6"(w803) -> ()
      }
    }
    n263 = call "PADMINI_STOP_ALL.vi"("Enum"=enum16{"Read", "Write"}."Read") -> ("Boolean 2"=w668:bool)  [unwired: 9 in, 1 out]
    n264 = local read "stop"() -> (w667:bool)
    n265 = Or(x=w667, y=w668) -> (x .or. y?=w666:bool)
    n266 = Wait (ms)(milliseconds to wait=u32 50) -> ()  [unwired: 1 out]
  }
  n267 = call <vilib>:"Clear Errors.vi"("error in (no error)"=w104) -> ("error out"=w105:errorcluster)  [unwired: 5 in, 1 out]
  n268 = call <vilib>:"Clear Errors.vi"("error in (no error)"=w113) -> ("error out"=w115:errorcluster)  [unwired: 5 in, 1 out]
  n269 = call <vilib>:"Clear Errors.vi"("error in (no error)"=w86) -> ("error out"=w85:errorcluster)  [unwired: 5 in, 1 out]
  n270 = call <vilib>:"Clear Errors.vi"("error in (no error)"=w60) -> ("error out"=w61:errorcluster)  [unwired: 5 in, 1 out]
  n271 = call <vilib>:"disconnect.vi"("error in (no error)"=w105, "S7 Connection in"=w103) -> ("error out"=w102:errorcluster)  [unwired: 8 in, 1 out]
  n272 = call <vilib>:"disconnect.vi"("error in (no error)"=w115, "S7 Connection in"=w114) -> ("error out"=w101:errorcluster)  [unwired: 8 in, 1 out]
  n273 = call <vilib>:"disconnect.vi"("error in (no error)"=w85, "S7 Connection in"=w87) -> ("error out"=w57:errorcluster)  [unwired: 8 in, 1 out]
  n274 = call <vilib>:"disconnect.vi"("error in (no error)"=w61, "S7 Connection in"=w59) -> ("error out"=w56:errorcluster)  [unwired: 8 in, 1 out]
  n275 = Merge Errors(w101, w102, w57, w56) -> (w100:errorcluster)
  n276 = call <vilib>:"Clear Errors.vi"("error in (no error)"=w38) -> ("error out"=w39:errorcluster)  [unwired: 5 in, 1 out]
  n277 = call <vilib>:"disconnect.vi"("error in (no error)"=w39, "S7 Connection in"=w37) -> ("error out"=w3:errorcluster)  [unwired: 8 in, 1 out]
  n278 = call <vilib>:"Clear Errors.vi"("error in (no error)"=w160) -> ("error out"=w145:errorcluster)  [unwired: 5 in, 1 out]
  n279 = call <vilib>:"disconnect.vi"("error in (no error)"=w145, "S7 Connection in"=w144) -> ("error out"=w143:errorcluster)  [unwired: 8 in, 1 out]
  n280 = call <vilib>:"Clear Errors.vi"("error in (no error)"=w5) -> ("error out"=w6:errorcluster)  [unwired: 5 in, 1 out]
  n281 = call <vilib>:"disconnect.vi"("error in (no error)"=w6, "S7 Connection in"=w4) -> ("error out"=w1:errorcluster)  [unwired: 8 in, 1 out]
  n282 = Merge Errors(w3, w1) -> (w2:errorcluster)
  n283 = Merge Errors(w143, w100, w2) -> (w165:errorcluster)
  n284 = call <vilib>:"Simple Error Handler.vi"("error in (no error)"=w165) -> ("error out"=w164:errorcluster)  [unwired: 4 in, 4 out]
  n285 = call <vilib>:"Clear Errors.vi"("error in (no error)"=w164) -> ("error out"=w163:errorcluster)  [unwired: 5 in, 1 out]
  n286 = invoke class="VI" method="FP.Close"(error in=w163) -> (error out=→"error out":errorcluster)  [unwired: 2 in, 2 out]
